vi "Drive Config.vi"(8 "error in (no error)":errorcluster, 11 "FileConfig in":refnum<class "FileConfig.lvclass">) -> (0 "error out":errorcluster, 1 "IDs found?":bool, 2 "Robot Drivetrain Data":T1={"Right"={"Talon"=0, "Victor1"=0, "Victor2"=0}, "Left"={"Talon"=0, "Victor1"=0, "Victor2"=0}, "Drive Velocity Low Gear"={"P"=0.0, "I"=0.0, "D"=0.0, "F"=0.0, "integralZone"=0.0, "allowableClosedLoopError"=0, "maxIntegralAccumulator"=0.0, "closedLoopPeakOutput"=1.0, "closedLoopPeriod"=1}, "Drive Velocity High Gear"={"P"=0.0, "I"=0.0, "D"=0.0, "F"=0.0, "integralZone"=0.0, "allowableClosedLoopError"=0, "maxIntegralAccumulator"=0.0, "closedLoopPeakOutput"=1.0, "closedLoopPeriod"=1}, "Drive Motion Magic Primary Low Gear"={"P"=0.0, "I"=0.0, "D"=0.0, "F"=0.0, "integralZone"=0.0, "allowableClosedLoopError"=0, "maxIntegralAccumulator"=0.0, "closedLoopPeakOutput"=1.0, "closedLoopPeriod"=1}, "Drive Motion Magic Primary High Gear"={"P"=0.0, "I"=0.0, "D"=0.0, "F"=0.0, "integralZone"=0.0, "allowableClosedLoopError"=0, "maxIntegralAccumulator"=0.0, "closedLoopPeakOutput"=1.0, "closedLoopPeriod"=1}, "Drive Motion Magic Secondary Low Gear"={"P"=0.0, "I"=0.0, "D"=0.0, "F"=0.0, "integralZone"=0.0, "allowableClosedLoopError"=0, "maxIntegralAccumulator"=0.0, "closedLoopPeakOutput"=1.0, "closedLoopPeriod"=1}, "Drive Motion Magic Secondary High Gear"={"P"=0.0, "I"=0.0, "D"=0.0, "F"=0.0, "integralZone"=0.0, "allowableClosedLoopError"=0, "maxIntegralAccumulator"=0.0, "closedLoopPeakOutput"=1.0, "closedLoopPeriod"=1}, "Drive Right Invert"=FALSE, "Drive Right Sensor Phase"=FALSE, "Drive Left Invert"=FALSE, "Drive Left Sensor Phase"=FALSE, "Low Gear Max Velocity"=0, "High Gear Max Velocity"=0, "Motion Magic Low Gear Max Velocity"=0, "Motion Magic Low Gear Max Acceleration"=0, "Motion Magic High Gear Max Velocity"=0, "Motion Magic High Gear Max Acceleration"=0}, 3 "FileConfig out":refnum<class "FileConfig.lvclass">, 4 "PIDFs found":bool, 5 "File Found?":bool)   [LabVIEW 2019, in "Config.lvlib" / "FileConfig.lvclass"]
doc: "Use this VI to configure the drive. It will return both if it found the slots, as well as the PIDF values."
uses:
  FileConfig.lvclass
  Config.lvclass
  Drive/Pod Drive/Controls/Pod.ctl
  Config/Controls/Drivetrain Data.ctl
  <vilib>/Rock Robotics/WPI/ThirdParty/Phoenix-LabVIEW/Motor Controller/Controls/CTRE_Phoenix_MotorControl_SlotStructure.ctl
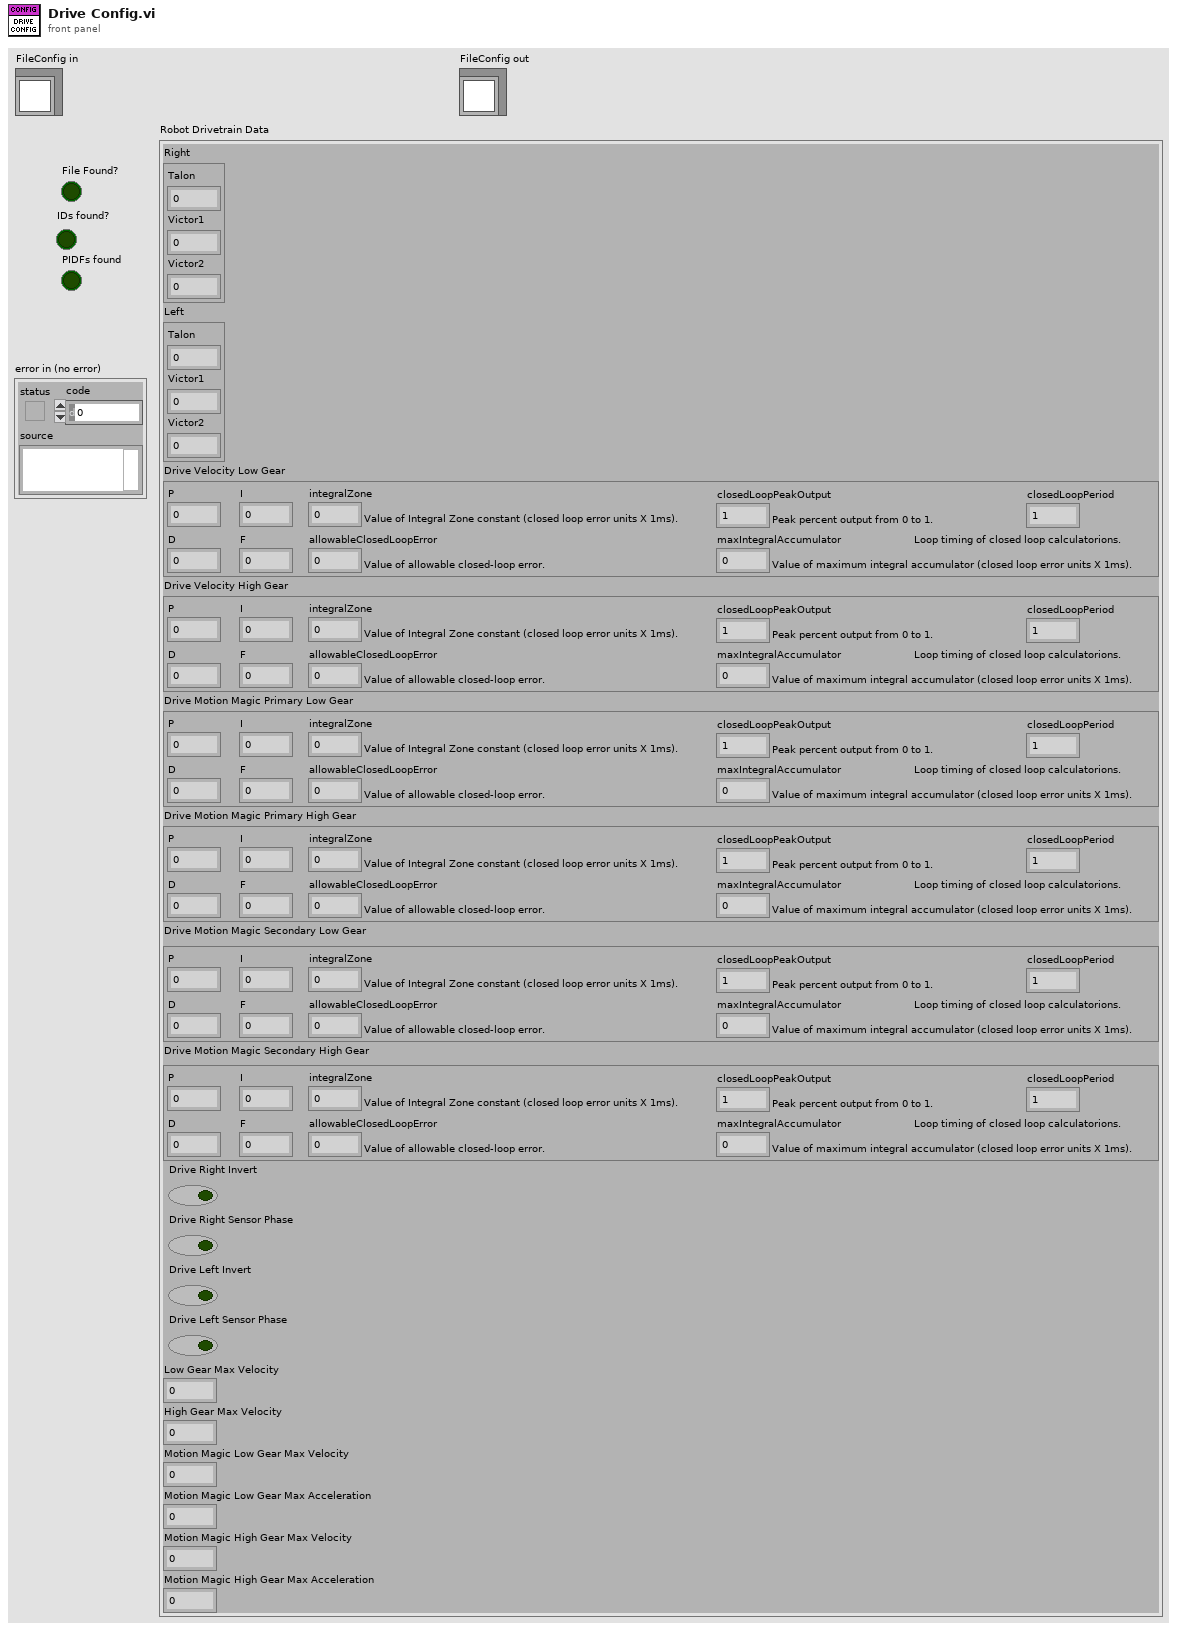
[diagram p1: front panel]
types:
  T1 = typedef "Config.lvlib/Config.lvclass/Drivetrain Data.ctl" = cluster{"Right":T2, "Left":T2, "Drive Velocity Low Gear":T3, "Drive Velocity High Gear":T3, "Drive Motion Magic Primary Low Gear":T3, "Drive Motion Magic Primary High Gear":T3, "Drive Motion Magic Secondary Low Gear":T3, "Drive Motion Magic Secondary High Gear":T3, "Drive Right Invert":bool, "Drive Right Sensor Phase":bool, "Drive Left Invert":bool, "Drive Left Sensor Phase":bool, "Low Gear Max Velocity":u32, "High Gear Max Velocity":u32, "Motion Magic Low Gear Max Velocity":u32, "Motion Magic Low Gear Max Acceleration":u32, "Motion Magic High Gear Max Velocity":u32, "Motion Magic High Gear Max Acceleration":u32}
  T2 = typedef "Drive.lvlib/Pod Drive.lvclass/Pod.ctl" = cluster{"Talon":u8, "Victor1":u8, "Victor2":u8}
  T3 = typedef "CTRE_Phoenix_MotorControl_SlotStructure.ctl" = cluster{"P":dbl, "I":dbl, "D":dbl, "F":dbl, "integralZone":dbl, "allowableClosedLoopError":i32, "maxIntegralAccumulator":dbl, "closedLoopPeakOutput":dbl, "closedLoopPeriod":i32}
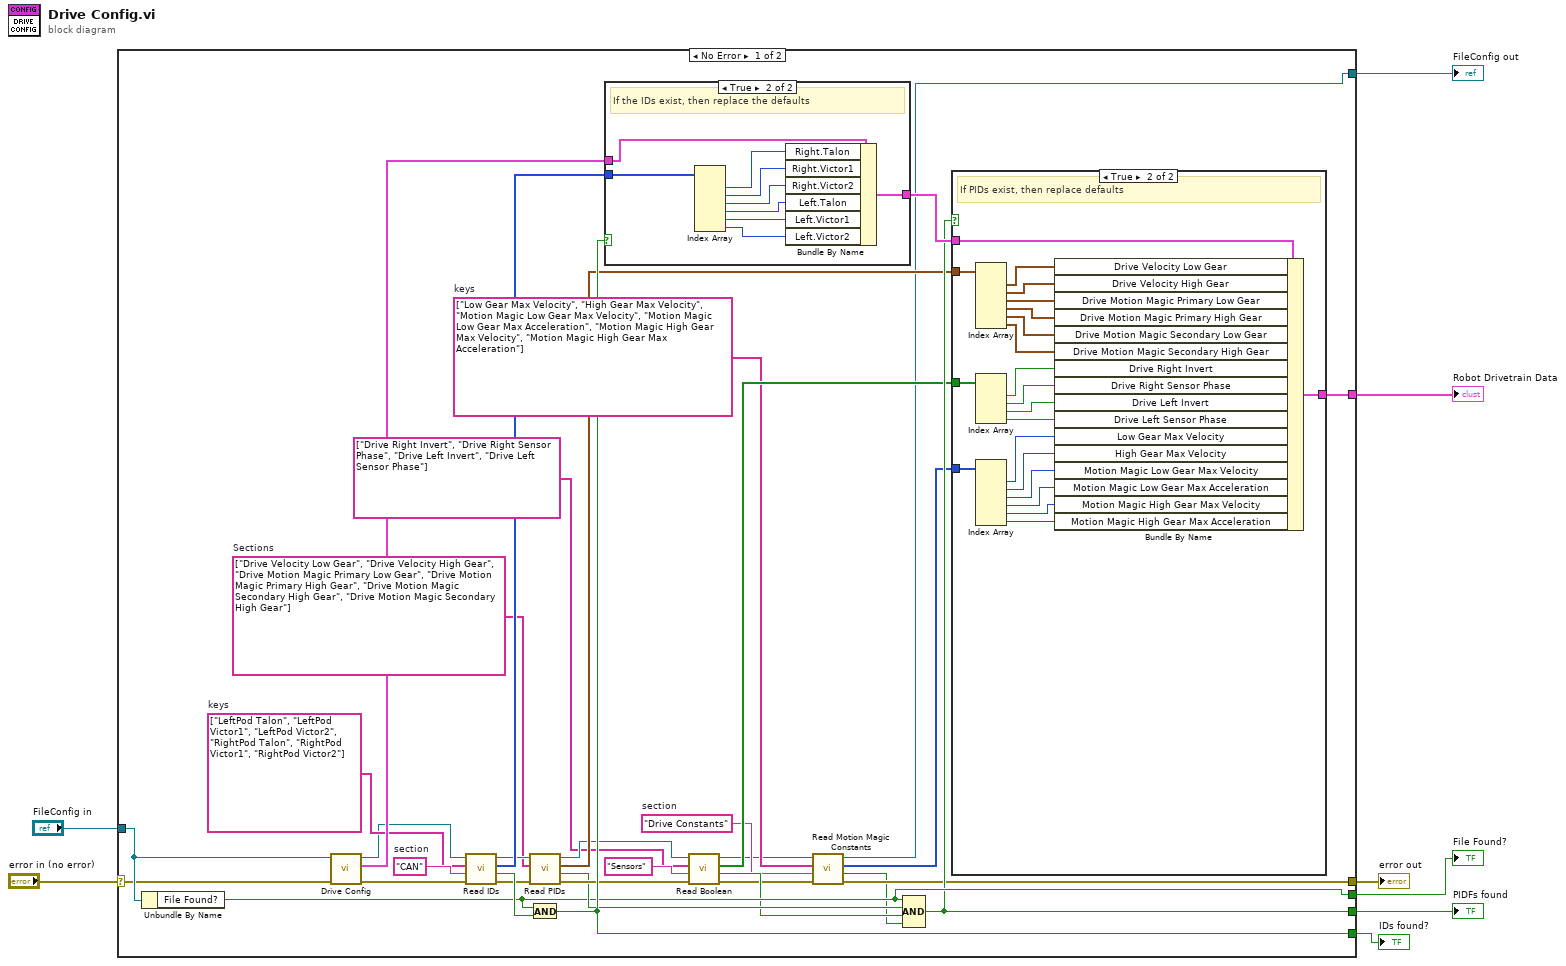
[diagram p0: block diagram]
diagram:
  n1 = case shown="No Error" "error in (no error)" {
    selector: "error in (no error)" -> [w27 w74]
    tunnel: [w11 w74] -> w8
    tunnel: [w24 _] -> w7
    tunnel: [w13 w75] -> w6
    tunnel: "FileConfig in" -> [w29 w75]
    tunnel: [w37 _] -> w3
    tunnel: [w30 _] -> w2
    tunnel: [w23 _] -> w1
    frame No Error {
      w16 = string[] ["Low Gear Max Velocity", "High Gear Max Velocity", "Motion Magic Low Gear Max Velocity", "Motion Magic Low Gear Max Acceleration", "Motion Magic High Gear Max Velocity", "Motion Magic High Gear Max Acceleration"]  # keys
      w15 = "Drive Constants"  # section
      w32 = string[] ["Drive Velocity Low Gear", "Drive Velocity High Gear", "Drive Motion Magic Primary Low Gear", "Drive Motion Magic Primary High Gear", "Drive Motion Magic Secondary High Gear", "Drive Motion Magic Secondary High Gear"]  # Sections
      w39 = string[] ["LeftPod Talon", "LeftPod Victor1", "LeftPod Victor2", "RightPod Talon", "RightPod Victor1", "RightPod Victor2"]  # keys
      w40 = "CAN"  # section
      n2 = Unbundle By Name(w29) -> ("File Found?"=w30:bool)
      n3 = call-parent "Drive Config.vi"("error in (no error)"=w27, "Config in"=w29) -> ("error out"=w26:errorcluster, "Robot Drivetrain Data"=w41:T1, "Config out"=w28:refnum<class "FileConfig.lvclass">)  [unwired: 4 in, 3 out]
      n4 = call "Read IDs.vi"("error in (no error)"=w26, "section"=w40, "keys"=w39, "FileConfig in"=w28) -> ("error out"=w34:errorcluster, "Found?"=w36:bool, "Found IDs"=w38:u8[], "FileConfig out"=w35:refnum<class "FileConfig.lvclass">)  [unwired: 4 in]
      n5 = call "Read PIDs.vi"("error in (no error)"=w34, "PID Sections to read"=w32, "FileConfig in"=w35) -> ("error out"=w33:errorcluster, "Found?"=w31:bool, "PIDF Array"=w22:T3[], "FileConfig out"=w21:refnum<class "FileConfig.lvclass">)  [unwired: 5 in]
      n6 = And(x=w30, y=w36) -> (x .and. y?=w37:bool)
      n7 = case shown="True" w37 {
        tunnel: w41 -> [w64 w73]
        tunnel: [w64 w72] -> w25
        tunnel: w38 -> [_ w71]
        frame False {
        }
        frame True {
          # "If the IDs exist, then replace the defaults"
          n8 = Index Array(array=w71) -> (element #1=w70:u8, element #2=w69:u8, element #3=w68:u8, element #4=w67:u8, element #5=w66:u8, element #6=w65:u8)  [unwired: 6 in]
          n9 = Bundle By Name(cluster=w73, "Right.Talon"=w70, "Right.Victor1"=w69, "Right.Victor2"=w68, "Left.Talon"=w67, "Left.Victor1"=w66, "Left.Victor2"=w65) -> (w72:T1)
        }
      }
      n10 = call "Read Boolean.vi"("error in (no error)"=w33, "section"="Sensors", "keys"=string[] ["Drive Right Invert", "Drive Right Sensor Phase", "Drive Left Invert", "Drive Left Sensor Phase"], "FileConfig in"=w21) -> ("error out"=w12:errorcluster, "Found?"=w20:bool, "Found Booleans"=w19:bool[], "FileConfig out"=w14:refnum<class "FileConfig.lvclass">)  [unwired: 4 in]
      n11 = call "Read Motion Magic Constants.vi"("error in (no error)"=w12, "section"=w15, "keys"=w16, "FileConfig in"=w14) -> ("error out"=w11:errorcluster, "Found?"=w10:bool, "Found Constants"=w9:u32[], "FileConfig out"=w13:refnum<class "FileConfig.lvclass">)  [unwired: 4 in]
      n12 = Compound Arithmetic op=AND(w30, w31, w20, w10) -> (w23:bool)
      n13 = case shown="True" w23 {
        tunnel: w25 -> [w42 w63]
        tunnel: [w42 w62] -> w24
        tunnel: w22 -> [_ w61]
        tunnel: w19 -> [_ w56]
        tunnel: w9 -> [_ w49]
        frame False {
        }
        frame True {
          # "If PIDs exist, then replace defaults"
          n14 = Index Array(array=w61) -> (element #1=w60:T3, element #2=w59:T3, element #3=w58:T3, element #4=w57:T3, element #5=w51:T3, element #6=w50:T3)  [unwired: 6 in]
          n15 = Index Array(array=w56) -> (element #1=w55:bool, element #2=w54:bool, element #3=w53:bool, element #4=w52:bool)  [unwired: 4 in]
          n16 = Index Array(array=w49) -> (element #1=w48:u32, element #2=w47:u32, element #3=w46:u32, element #4=w45:u32, element #5=w44:u32, element #6=w43:u32)  [unwired: 6 in]
          n17 = Bundle By Name(cluster=w63, "Drive Velocity Low Gear"=w60, "Drive Velocity High Gear"=w59, "Drive Motion Magic Primary Low Gear"=w58, "Drive Motion Magic Primary High Gear"=w57, "Drive Motion Magic Secondary Low Gear"=w51, "Drive Motion Magic Secondary High Gear"=w50, "Drive Right Invert"=w55, "Drive Right Sensor Phase"=w54, "Drive Left Invert"=w53, "Drive Left Sensor Phase"=w52, "Low Gear Max Velocity"=w48, "High Gear Max Velocity"=w47, "Motion Magic Low Gear Max Velocity"=w46, "Motion Magic Low Gear Max Acceleration"=w45, "Motion Magic High Gear Max Velocity"=w44, "Motion Magic High Gear Max Acceleration"=w43) -> (w62:T1)
        }
      }
    }
    frame Error {
    }
  }
  "error out" <- w8
  "FileConfig out" <- w6
  "Robot Drivetrain Data" <- w7
  "File Found?" <- w2
  "IDs found?" <- w3
  "PIDFs found" <- w1
